vi "LVClass_HasoEngine Compute Internal slopes.vi"(0 "HasoEngine in":refnum<class "HasoEngine.lvclass">, 7 "Image.lvclass":refnum<class "Image.lvclass">, 9 "learn_from_trimmer":bool, 11 "error in (no error)":errorcluster, 12 "check_calibration_checksum":bool) -> (4 "HasoEngine out":refnum<class "HasoEngine.lvclass">, 6 "HasoSlopes (dup)":refnum<class "HasoSlopes.lvclass">, 8 "Image (dup)":refnum<class "Image.lvclass">, 14 "trimmer_quality":sgl, 15 "error out":errorcluster)   [LabVIEW 2020, in "HasoEngine.lvclass"]
doc: "Compute HasoSlopes. Please check that computation preferences have been set,\nand alignment step is completed.\n\n--------------------------------------------------------------------------------\n\n<B>HasoEngineIn </B> : HasoEngine object.\n<B>HasoEngineOut </B> : HasoEngine object.\n<B>HasoSlopes </B> : Computed Hasoslopes.\n<B>image </B> : Input image object.\n<B>align_from_trimmer </B> : If True, a possible mis-alignement is corrected by correlating the observed\n high-frequency aberrations. with a pre-calibrated map (trimmer). \n WARNING : The results may be distorted if the analyzed wavefront presents\n high-frequency aberrations or if the illuminated surface area on the sensor\n is too small (< 30%).\n<B>trimmer_quality </B> : If align_from_trimmer is true, correlation factor between the observed high-\n frequency aberrations and the pre-calibrated map.\n<B>ErrorIn </B> : Error\n<B>ErrorOut </B> : Error\n\n--------------------------------------------------------------------------------"
uses:
  HasoEngine.lvclass
  Image/Image.lvclass
  HasoSlopes/HasoSlopes.lvclass
  HasoEngine.lvclass/HasoEngine.ctl
  Image/LVClass_Image read Image Compat ptr.vi
  HasoSlopes/LVClass_HasoSlopes Read HasoSlopes _ property.vi
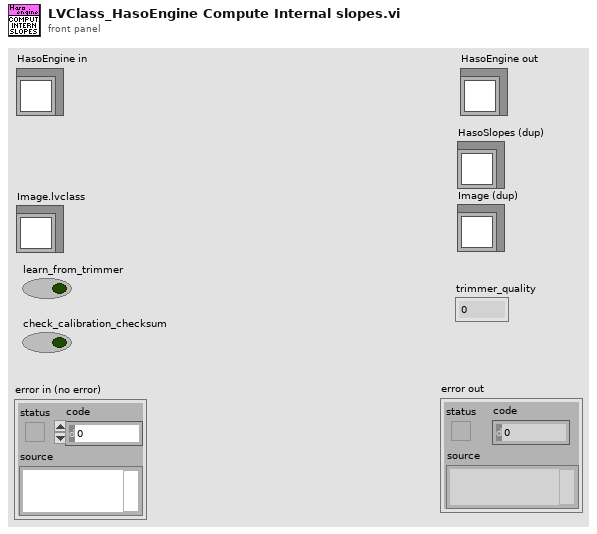
[diagram p1: front panel]
types:
  T1 = typedef "ClassID.ctl" = i64
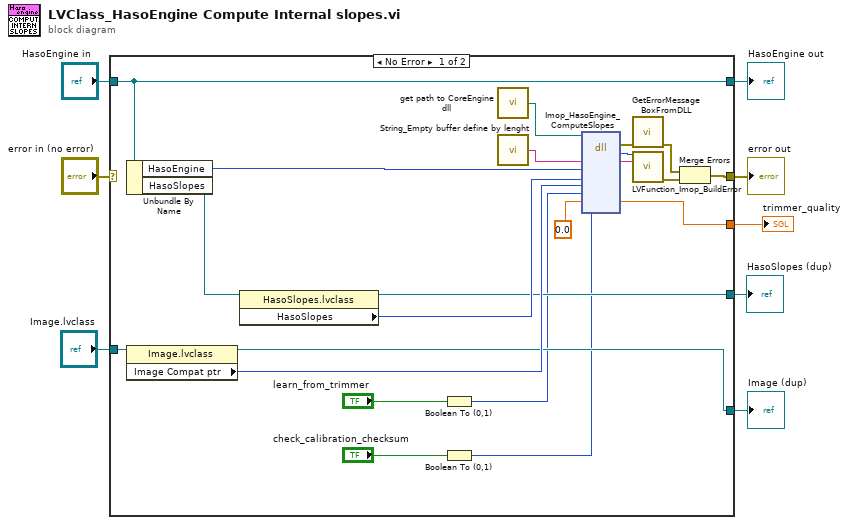
[diagram p0: block diagram]
diagram:
  n1 = case shown="No Error" "error in (no error)" {
    selector: "error in (no error)" -> [_ w32]
    tunnel: "HasoEngine in" -> [w17 w33]
    tunnel: [w17 w33] -> w5
    tunnel: [w12 w32] -> w6
    tunnel: "Image.lvclass" -> [w25 w31]
    tunnel: [w21 _] -> w3
    tunnel: [w20 w31] -> w2
    tunnel: [w11 _] -> w1
    frame No Error {
      n2 = Unbundle By Name(w17) -> ("HasoEngine"=w16:T1, "HasoSlopes"=w15:refnum<class "HasoSlopes.lvclass">)
      n3 = property class="Image.lvclass"(reference=w25) -> (reference out=w20:refnum<class "Image.lvclass">, "Image Compat ptr"=w23:T1)  [unwired: 1 in, 1 out]
      n4 = property class="HasoSlopes.lvclass"(reference=w15) -> (reference out=w21:refnum<class "HasoSlopes.lvclass">, "HasoSlopes"=w24:T1)  [unwired: 1 in, 1 out]
      n5 = Boolean To (0,1)(Boolean="learn_from_trimmer") -> (0, 1=w18:i16)
      n6 = Boolean To (0,1)(Boolean="check_calibration_checksum") -> (0, 1=w9:i16)
      n7 = call "get path to CoreEngine dll.vi"() -> ("path to wavekit library"=w27:path)  [unwired: 14 in, 1 out]
      n8 = call "String_Empty buffer define by lenght.vi"() -> ("Empty buffer"=w30:string)  [unwired: 1 in]
      n9 = dll-call lib="D:/2_trunk/Soft_haso/ImOpCoreEngine4_LV2011/DLLs/ImopEngine4_vc100.dll" fn="Imop_HasoEngine_ComputeSlopes"(path in=w27, "message"=w30, "Slopes Engine"=w16, "Data Slopes"=w24, "Image"=w23, "learn_from_trimmer"=w18, "trimmer_quality"=sgl 0.0, "check_calibration_checksum"=w9) -> (error out=w26:errorcluster, "return type"=w28:i32, "message"=w29:string, "trimmer_quality"=w11:sgl)  [unwired: 7 in, 1 out]
      n10 = call "GetErrorMessageBoxFromDLL.vi"("error IN"=w26) -> ("error OUT"=w14:errorcluster)  [unwired: 10 in]
      n11 = call "LVFunction_Imop_BuildError.vi"("code"=w28, "String to Prepend to source (\"\")"=w29) -> ("error out"=w13:errorcluster)  [unwired: 13 in]
      n12 = Merge Errors(w14, w13) -> (w12:errorcluster)
    }
    frame Error {
    }
  }
  "error out" <- w6
  "HasoEngine out" <- w5
  "HasoSlopes (dup)" <- w3
  "Image (dup)" <- w2
  "trimmer_quality" <- w1
